vi "NI VeriStand - Remove Error.vi"(8 "error in (no error)":errorcluster, 10 "Error ID":string, 11 "Node Ref in":T1 format="%.0x") -> (0 "error out":errorcluster, 3 "Node Ref out":T1=18446744073709551615 format="%.0x")   [LabVIEW 2026, in "Custom Devices Storage.lvlib"]
uses:
  Custom Devices Storage.lvlib
  <vilib>/NI VeriStand/Custom Device API/Custom Device Item Ref.ctl
  <vilib>/NI VeriStand/Custom Device API/Custom Device API.lvlib
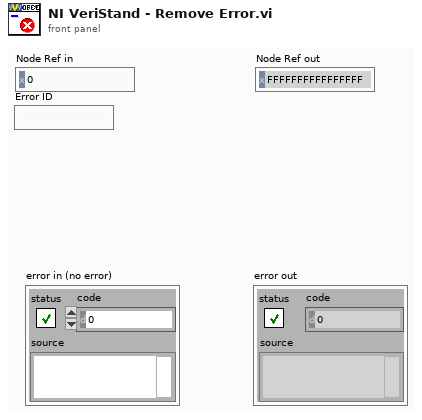
[diagram p1: front panel]
types:
  T1 = typedef "Custom Device API.lvlib/Custom Device Item Ref.ctl" = u64
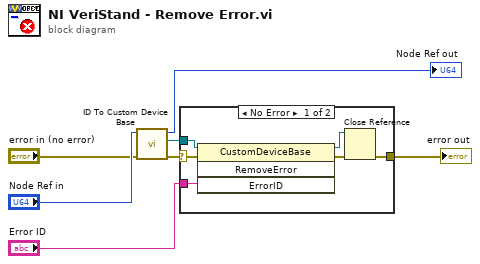
[diagram p0: block diagram]
diagram:
  n1 = call "ID To Custom Device Base.vi"("error in (no error)"="error in (no error)", "ID in"="Node Ref in") -> ("error out"=w5:errorcluster, "BaseNode"=w4:refnum<k39>, "ID out"=→"Node Ref out":u64)  [unwired: 7 in]
  n2 = case shown="No Error" w5 {
    selector: w5 -> [w12 w14]
    tunnel: w4 -> [w13 _]
    tunnel: "Error ID" -> [w11 _]
    tunnel: [w8 w14] -> w2
    frame No Error {
      n3 = invoke class="CustomDeviceBase" method="RemoveError"(reference=w13, error in=w12, "ErrorID"=w11) -> (reference out=w9:refnum<k39>, error out=w10:errorcluster)  [unwired: 1 in, 2 out]
      n4 = Close Reference(reference=w9, error in (no error)=w10) -> (error out=w8:errorcluster)
    }
    frame Error {
    }
  }
  "error out" <- w2
